vi "Stop Connection Handler.vi"(8 "error in (no error)":errorcluster, 11 "TCPConnectionHandler in":refnum<class "ConnectionHandler.lvclass">) -> (0 "error out":errorcluster, 3 "TCPConnectionHandler out":refnum<class "ConnectionHandler.lvclass">)   [LabVIEW 2013, in "MQTT_Connection.lvlib" / "ConnectionHandler.lvclass"]
uses:
  ConnectionHandler.lvclass
  ConnectionHandler.lvclass/ConnectionHandler.ctl
panel:
  out "timed out?":bool
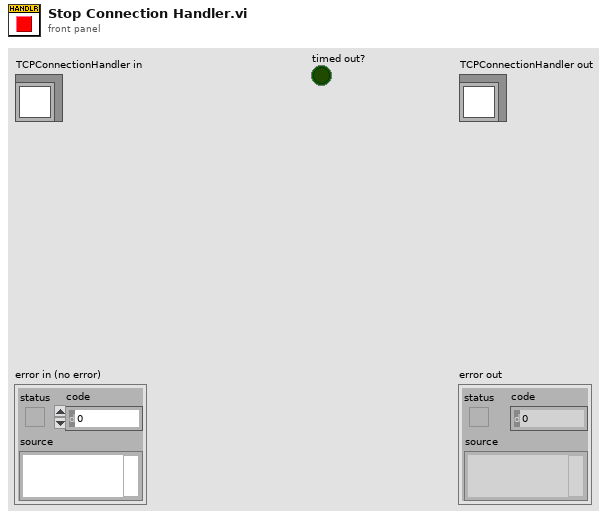
[diagram p1: front panel]
types:
  T1 = typedef "MQTT_Connection.lvlib/ConnectionHandler.lvclass/Public Events -- Cluster.ctl" = cluster{"NbConnections":refnum<user-event>}
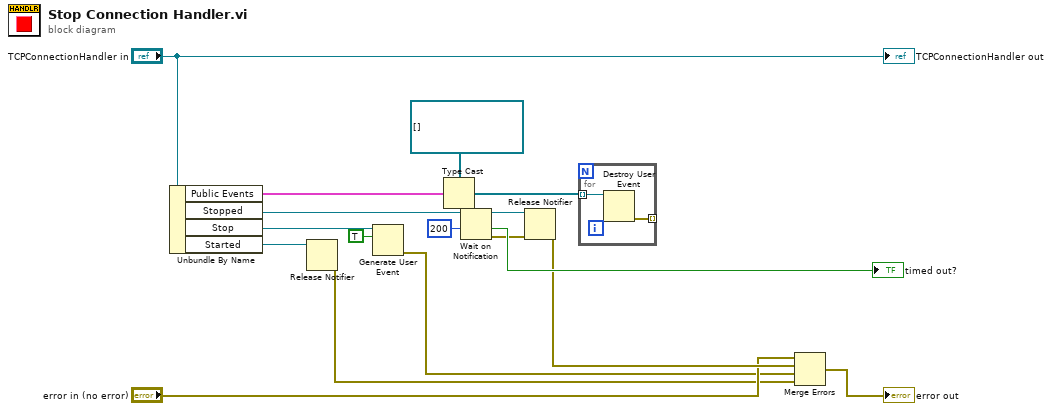
[diagram p0: block diagram]
diagram:
  n1 = Unbundle By Name("TCPConnectionHandler in") -> ("Public Events"=w2:T1, "Stopped"=w13:refnum<notifier>, "Stop"=w15:refnum<user-event>, "Started"=w5:refnum<notifier>)
  n2 = Release Notifier(notifier=w5) -> (error out=w4:errorcluster)  [unwired: 2 in, 2 out]
  n3 = Generate User Event(user event=w15, event data cluster=TRUE ("event data")) -> (error out=w6:errorcluster)  [unwired: 2 in, 1 out]
  n4 = Type Cast(type=refnum<user-event>[] [], x=w2) -> (*(type *) &x=w1:refnum<user-event>[])
  n5 = Wait on Notification(notifier=w13, timeout in ms (-1)=200) -> (notifier out=w10:refnum<notifier>, timed out?=→"timed out?":bool, error out=w11:errorcluster)  [unwired: 2 in, 1 out]
  n6 = Release Notifier(notifier=w10, error in (no error)=w11) -> (error out=w9:errorcluster)  [unwired: 1 in, 2 out]
  n7 = for {
    tunnel: w1 -> [w19] mode=indexing
    tunnel: [w18] -> _ mode=indexing
    n8 = Destroy User Event(user event=w19) -> (error out=w18:errorcluster)  [unwired: 1 in]
  }
  n9 = Merge Errors("error in (no error)", w9, w6, w4) -> (→"error out":errorcluster)
  "TCPConnectionHandler out" <- "TCPConnectionHandler in"
